vi "Write Ramp Current.vi"(8 "error in":errorcluster, 10 "Current_Ramp":dbl, 11 "6700C in":refnum<class "6700C.lvclass">) -> (0 "error out":errorcluster, 3 "6700C out":refnum<class "6700C.lvclass">)   [LabVIEW 2019, in "6700C.lvlib" / "6700C.lvclass"]
uses:
  Library/6700C.lvclass
  C:/Users/Public/Documents/Development/builds/Engine/Monitored Actor.lvlibp/Monitored Actor/Monitored Actor/Monitored Actor.lvclass
  builds/Engine/Monitored Actor.lvlibp/Monitored Actor/Monitored Actor/Read Actor Label.vi
  builds/Instruments/PowerSupply.lvlibp/Library/PowerSupply.lvclass
  <vilib>/ErrorRing/Error Ring.xnode
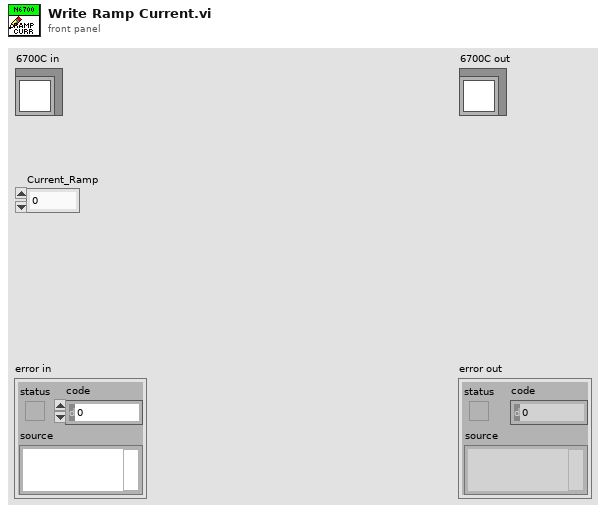
[diagram p1: front panel]
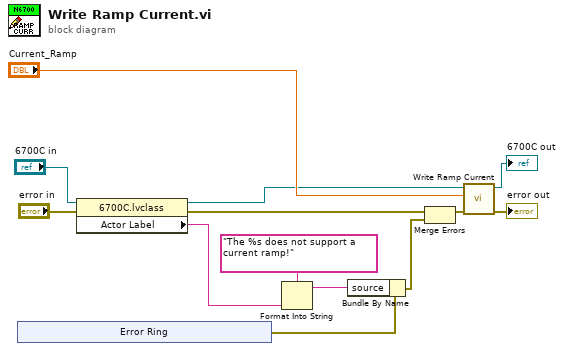
[diagram p0: block diagram]
diagram:
  n1 = xnode "Error Ring"() -> ("error out"=w1:errorcluster)
  n2 = property class="6700C.lvclass"(reference="6700C in", error in="error in") -> (reference out=w6:refnum<class "6700C.lvclass">, error out=w3:errorcluster, "Actor Label"=w10:string)
  n3 = Format Into String(format string="The %s does not support a current ramp!", w10) -> (resulting string=w9:string)  [unwired: 2 in, 1 out]
  n4 = Bundle By Name(cluster=w1, "source"=w9) -> (w2:errorcluster)
  n5 = Merge Errors(w3, w2) -> (w4:errorcluster)
  n6 = call-parent "Write Ramp Current.vi"("error in"=w4, "Current_Ramp"="Current_Ramp", "PowerSupply in"=w6) -> ("error out"=→"error out":errorcluster, "PowerSupply out"=→"6700C out":refnum<class "6700C.lvclass">)  [unwired: 7 in]
